vi "filter tags by type.vi"(10 "allowable types":T1[](array[typedef]), 11 "tags in":refnum<class "tag descriptor.lvclass">[](array[class])) -> (3 "filtered tags":refnum<class "tag descriptor.lvclass">[](array[class]))   [LabVIEW 2013, in "tag bus.lvlib" / "tag descriptor.lvclass"]
doc: "Filters a list of tags by type, eliminating all tags which do not match the desired set of types."
uses:
  tag descriptor.lvclass
  Data Type.ctl
  tag descriptor.lvclass/tag descriptor.ctl
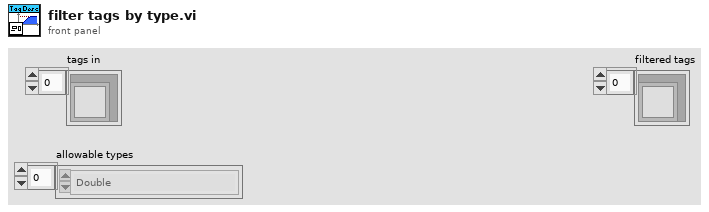
[diagram p1: front panel]
types:
  T1 = typedef "tag bus.lvlib/tag descriptor.lvclass/Data Type.ctl" = enum16{"Double", "Single", "I64", "I32", "I16", "I8", "U64", "U32", "U16", "U8", "Boolean", "String", "Array of Double", "Array of Single", "Array of I64", "Array of I32", "Array of I16", "Array of I8", "Array of U64", "Array of U32", "Array of U16", "Array of U8", "Array of Boolean", "Array of String"}
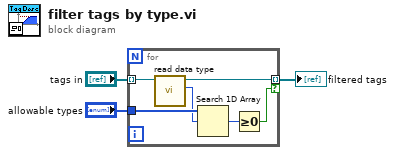
[diagram p0: block diagram]
diagram:
  n1 = for {
    tunnel: [w8] -> w3 mode=indexing if=w4
    tunnel: "tags in" -> [w9] mode=indexing
    tunnel: "allowable types" -> [w7]
    n2 = call "read data type.vi"("system tag in"=w9) -> ("data type"=w6:T1, "system tag out"=w8:refnum<class "tag descriptor.lvclass">)  [unwired: 8 in, 1 out]
    n3 = Search 1D Array(1D array=w7, element=w6) -> (index of element=w5:i32)  [unwired: 1 in]
    n4 = Greater Or Equal To 0?(x=w5) -> (x >= 0?=w4:bool)
  }
  "filtered tags" <- w3
